vi "SQL_Create.vi"(8 "error in (no error)":errorcluster, 10 "Ini Reference":T1, 11 "reference in":refnum<class "SQL.lvclass">) -> (0 "error out":errorcluster, 3 "reference out":refnum<class "SQL.lvclass">)   [LabVIEW 2012, in "SQL.lvclass"]
uses:
  SQL.lvclass
  <vilib>/Utility/config.llb/Config Data RefNum.ctl
  <vilib>/addons/database/Connection.llb/DB Tools Open Connec (String).vi
  <vilib>/addons/database/NI_Database_API.lvlib
  <vilib>/Utility/config.llb/NI_LVConfig.lvlib
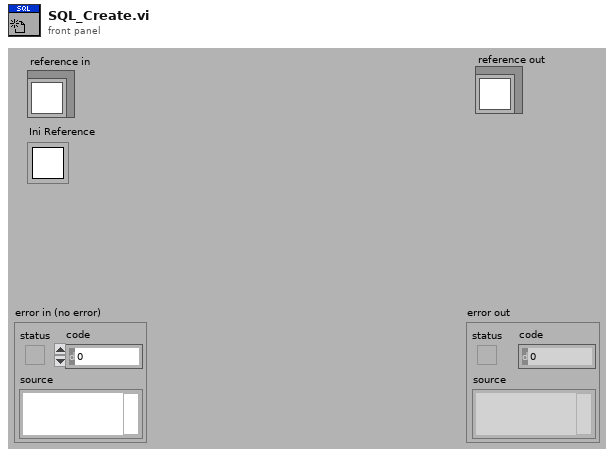
[diagram p1: front panel]
types:
  T1 = typedef "NI_LVConfig.lvlib/Config Data RefNum.ctl" = refnum<k1>
  T2 = typedef "SQL.lvclass/ObjectAttributes.ctl" = cluster{"DB Connection Reference":T3}
  T3 = typedef "NI_Database_API.lvlib/Conn ObjectReference.ctl" = refnum<k1>
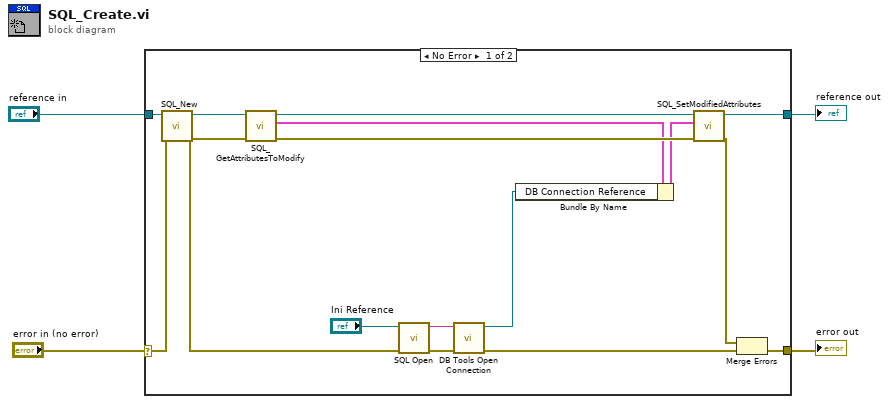
[diagram p0: block diagram]
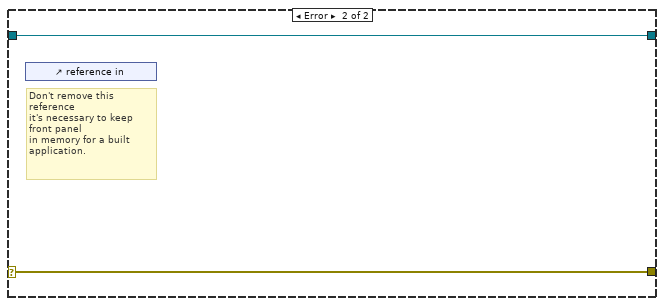
[diagram p2: hidden frame]
diagram:
  n1 = case shown="No Error" "error in (no error)" {
    selector: "error in (no error)" -> [w20 w22]
    tunnel: [w13 w22] -> w4
    tunnel: "reference in" -> [w15 w21]
    tunnel: [w16 w21] -> w2
    frame No Error {
      n2 = call "SQL_New.vi"("error in (no error)"=w20, "reference in"=w15) -> ("error out"=w11:errorcluster, "reference out"=w14:refnum<class "SQL.lvclass">)  [unwired: 6 in, 2 out]
      n3 = call "SQL_GetAttributesToModify.vi"("error in (no error)"=w11, "reference in"=w14) -> ("error out"=w19:errorcluster, "Attributes"=w6:T2, "reference out"=w18:refnum<class "SQL.lvclass">)  [unwired: 6 in, 1 out]
      n4 = call "SQL Open.vi"("error in (no error)"=w11, "Ini Reference"="Ini Reference") -> ("error out"=w10:errorcluster, "SQL Address"=w8:string)  [unwired: 8 in]
      n5 = call-poly <vilib>:"DB Tools Open Connection.vi"("error in (no error)"=w10, "connection information"=w8) -> ("error out"=w9:errorcluster, "connection reference"=w7:T3)  [unwired: 6 in]
      n6 = Bundle By Name(cluster=w6, "DB Connection Reference"=w7) -> (w17:T2)
      n7 = call "SQL_SetModifiedAttributes.vi"("error in (no error)"=w19, "Attributes"=w17, "reference in"=w18) -> ("error out"=w12:errorcluster, "reference out"=w16:refnum<class "SQL.lvclass">)  [unwired: 7 in]
      n8 = Merge Errors(w12, w9) -> (w13:errorcluster)
    }
    frame Error {
      # "Don't remove this reference\nit's necessary to keep front panel\nin memory for a built application."
      n9 = control-ref of="reference in"() -> ()  [unwired: 1 out]
    }
  }
  "error out" <- w4
  "reference out" <- w2
